vi "GE5565 Disable DMA Interrupt (Cluster) mod.vi"(4 "error in (no error)":errorcluster, 7 "VMIC reference in":T1) -> (0 "error out":errorcluster, 3 "VMIC reference out":T1)   [LabVIEW 2020, in "RefMem DMA Engine.lvlib"]
uses:
  RefMem DMA Engine.lvlib
  <vilib>/Instr/_visa.llb/Select Event Type.ctl
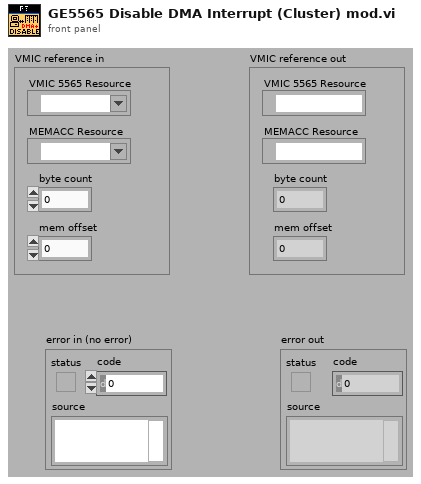
[diagram p1: front panel]
types:
  T1 = cluster{"VMIC 5565 Resource":refnum<visa-resource-name>, "MEMACC Resource":refnum<visa-resource-name>, "byte count":u32, "mem offset":u32}
  T2 = typedef "Select Event Type.ctl" = u32
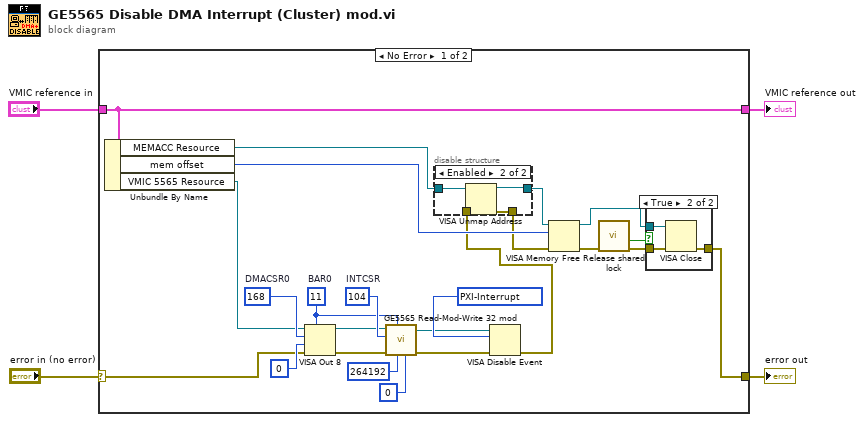
[diagram p0: block diagram]
diagram:
  n1 = case shown="No Error" "error in (no error)" {
    selector: "error in (no error)" -> [w26 w38]
    tunnel: "VMIC reference in" -> [w13 w39]
    tunnel: [w13 w39] -> w1
    tunnel: [w25 w38] -> w3
    frame No Error {
      w19 = u16 11  # BAR0
      w18 = T2 1073684514 items=["ServiceRequest"=1073684491, "Trigger"=3221168138, "Clear"=1073684493, "VXI-Signal"=1073684512, "VXI/VME-Interrupt"=3221168161, "VXI/VME-Sysfail"=1073684509, "VXI/VME-Sysreset"=1073684510, "GPIB-CIC"=1073684498, "GPIB-Talk"=1073684499, "GPIB-Listen"=1073684500, "PXI-Interrupt"=1073684514, "AllEnabled"=1073709055] ("Event Type")
      w24 = u32 104  # INTCSR
      w28 = u32 168  # DMACSR0
      n2 = Unbundle By Name(w13) -> ("MEMACC Resource"=w8:refnum<visa-resource-name>, "mem offset"=w14:u32, "VMIC 5565 Resource"=w15:refnum<visa-resource-name>)
      n3 = VISA Out 8(7:w19, 8:w26, 9:u8 0 ("value (0)"), 10:w28, 11:w15) -> (0:w20:errorcluster, 3:w21:refnum<visa-resource-name>)
      n4 = call "GE5565 Read-Mod-Write 32 mod.vi"("value"=u32 0, "inv bit mask"=u32 264192 ("value"), "address space (13: BAR2)"=w19, "error in (no error)"=w20, "offset (0)"=w24, "VISA resource name"=w21) -> ("error out"=w16:errorcluster, "VISA resource name out"=w17:refnum<visa-resource-name>)  [unwired: 4 in]
      n5 = VISA Disable Event(8:w16, 10:w18, 11:w17) -> (0:w6:errorcluster)  [unwired: 1 in, 1 out]
      n6 = disable-structure shown="Enabled" {
        disable-tunnel: w8 -> [w30 w33]
        disable-tunnel: [w30 w32] -> w7
        disable-tunnel: w6 -> [w29 _]
        disable-tunnel: [w29 w31] -> w5
        frame Disabled {
        }
        frame Enabled {
          n7 = VISA Unmap Address(11:w33) -> (0:w31:errorcluster, 3:w32:refnum<visa-resource-name>)  [unwired: 1 in]
        }
      }
      n8 = VISA Memory Free(8:w5, 10:w14, 11:w7) -> (0:w12:errorcluster, 3:w10:refnum<visa-resource-name>)
      n9 = call "Release shared lock.vi"("error in (no error)"=w12) -> ("error out"=w11:errorcluster, "Safe to delete"=w9:bool)  [unwired: 9 in]
      n10 = case shown="True" w9 {
        tunnel: [w34 w37] -> w25
        tunnel: w11 -> [w34 w36]
        tunnel: w10 -> [_ w35]
        frame False {
        }
        frame True {
          n11 = VISA Close(VISA resource name=w35, error in (no error)=w36) -> (error out=w37:errorcluster)
        }
      }
    }
    frame Error {
    }
  }
  "error out" <- w3
  "VMIC reference out" <- w1
